vi "Instruction Strings.vi"() -> (1 "output array":path[](array[path]), 3 "Array":string[](array[string]))   [LabVIEW 2024, in "Controller.lvlib" / "Controller.lvclass"]
uses:
  Controller/Controller.lvclass
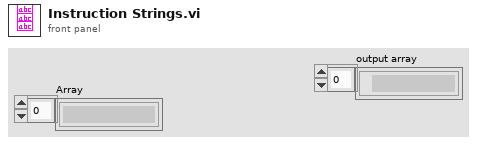
[diagram p1: front panel]
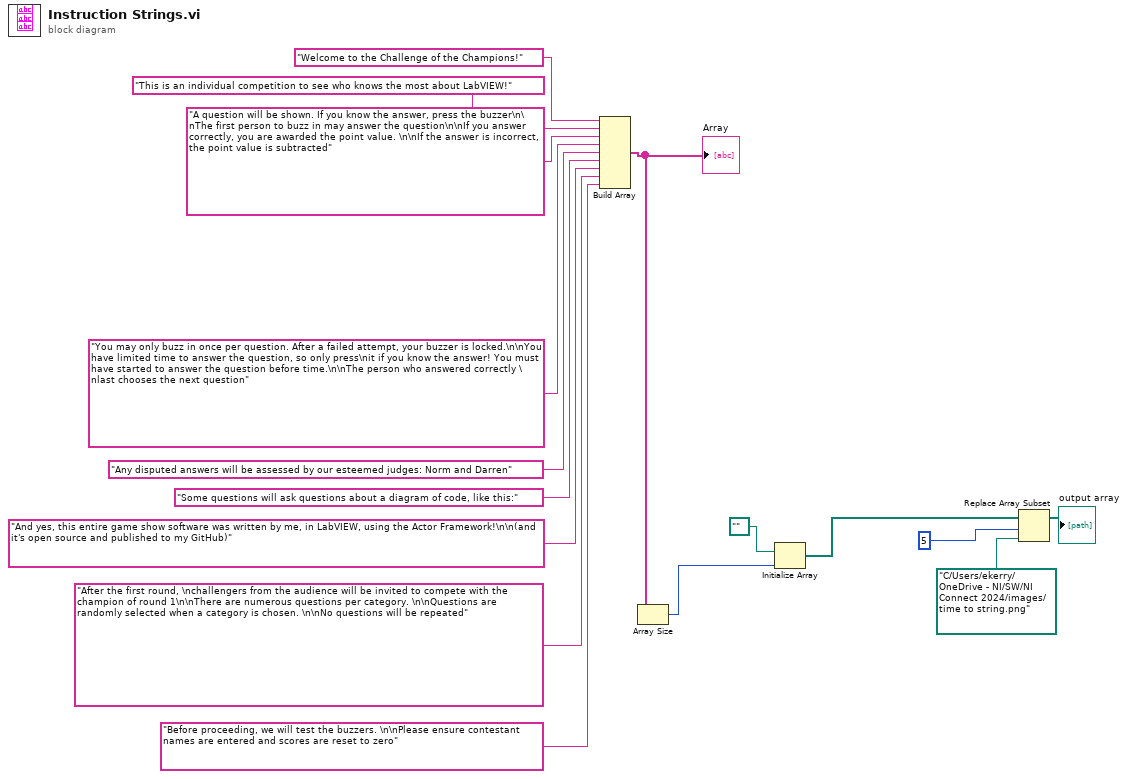
[diagram p0: block diagram]
diagram:
  n1 = Build Array("Welcome to the Challenge of the Champions!", "This is an individual competition to see who knows the most about LabVIEW!", "A question will be shown. If you know the answer, press the buzzer\n\nThe first person to buzz in may answer the question\n\nIf you answer correctly, you are awarded the point value. \n\nIf the answer is incorrect, the point value is subtracted", "You may only buzz in once per question. After a failed attempt, your buzzer is locked.\n\nYou have limited time to answer the question, so only press\nit if you know the answer! You must have started to answer the question before time.\n\nThe person who answered correctly \nlast chooses the next question" ("element"), "Any disputed answers will be assessed by our esteemed judges: Norm and Darren" ("element"), "Some questions will ask questions about a diagram of code, like this:" ("element"), "And yes, this entire game show software was written by me, in LabVIEW, using the Actor Framework!\n\n(and it's open source and published to my GitHub)" ("element"), "After the first round, \nchallengers from the audience will be invited to compete with the champion of round 1\n\nThere are numerous questions per category. \n\nQuestions are randomly selected when a category is chosen. \n\nNo questions will be repeated" ("element"), "Before proceeding, we will test the buzzers. \n\nPlease ensure contestant names are entered and scores are reset to zero" ("element")) -> (w2:string[])
  "Array" <- w2
  n2 = Array Size(array=w2) -> (size(s)=w4:i32)
  n3 = Initialize Array(path "" ("Image Path"), w4) -> (w3:path[])
  n4 = Replace Array Subset(array=w3, new element=path "C:/Users/ekerry/OneDrive - NI/SW/NI Connect 2024/images/time to string.png" ("new element/subarray"), index=5) -> (→"output array":path[])
